vi "SP Build Key Array for Config.vi"(8 "error in (no error)":errorcluster, 9 "S Parameter Test Parameters":T2={"Stimulus"={"Use Instrument Settings"=FALSE, "Blank Frequencies"=FALSE, "Sweep Type"=enum."Linear", "Sweep"={"Fstart"=500.0, "Fstop"=1500.0, "Units"=enum."MHz", "Points"=2}, "Power (dBm)"=999.0, "IFBW (Hz)"=-1.0, "Sweep Time (s)"=-1.0, "Calibration"={"State"=FALSE, "String"=""}}, "Measurement"={"Auto Select"=TRUE, "Data Source"=enum."VNA", "Ports"=2, "Parameters"=[]}, "De-Embed"={"De-Embed"=FALSE, "Adapters"=[]}, "Display"={"Lock Control"=FALSE, "Retain Settings"=TRUE, "Formatted Data"=FALSE, "Plot Orientation"=enum."Single", "Plot Controls"=[{"Trace Orientation"=enum."Overlay", "Frequency"={"Change Frequency"=FALSE, "Start"=500.0, "Stop"=1500.0, "Units"=enum."MHz"}, "Markers"=[], "Traces"=[]}, {"Trace Orientation"=enum."Overlay", "Frequency"={"Change Frequency"=FALSE, "Start"=500.0, "Stop"=1500.0, "Units"=enum."MHz"}, "Markers"=[], "Traces"=[]}, {"Trace Orientation"=enum."Overlay", "Frequency"={"Change Frequency"=FALSE, "Start"=500.0, "Stop"=1500.0, "Units"=enum."MHz"}, "Markers"=[], "Traces"=[]}, {"Trace Orientation"=enum."Overlay", "Frequency"={"Change Frequency"=FALSE, "Start"=500.0, "Stop"=1500.0, "Units"=enum."MHz"}, "Markers"=[], "Traces"=[]}]}, "Limits"=[], "Filter Limits"=[]} {"Filter Limits"."Parameter"."Stimulus Port" min=1 step=1; "Filter Limits"."Parameter"."Response Port" min=1 step=1; "Filter Limits"."Passband"."Bandwidth Attn" format="%.3g"; "Filter Limits"."Passband"."Stop/Span" format="%.3g"; "Filter Limits"."Passband"."Start/Center" format="%.3g"; "Measurement"."Parameters"."Channel" min=0 max=32 step=1; "Measurement"."Parameters"."Parameter"."Stimulus Port" min=1 step=1; "Measurement"."Parameters"."Parameter"."Response Port" min=1 step=1; "Limits"."Parameter"."Stimulus Port" min=1 step=1; "Limits"."Parameter"."Response Port" min=1 step=1; "Stimulus"."Sweep Time (s)" format="%.3g"; "Display"."Plot Controls"."Traces"."Reference" format="%#.2g"; "Display"."Plot Controls"."Traces"."Display Data" items=["Data", "Memory", "Data/Memory"]; "Display"."Plot Controls"."Traces"."Format" items=["Log Mag", "Phase", "Expanded Phase", "Delay", "Smith", "Polar", "Lin Mag", "SWR", "Loss", "Real", "Imaginary"]; "Display"."Plot Controls"."Traces"."Scale" min=0.001 step=1.0 format="%#.2g"; "Display"."Plot Controls"."Traces"."Position" min=0.0 max=10.0; "Display"."Plot Controls"."Frequency"."Stop" format="%.3g"; "Display"."Plot Controls"."Frequency"."Start" format="%.3g"}, 10 "Key Array In":T33, 11 "Connection Refnum":T1) -> (0 "error out":errorcluster, 1 "$$INITCODE$$":string, 2 "Key Array Out":T33, 3 "Connection Refnum":T1)   [LabVIEW 2011]
uses:
  ITK EXT/utils/keyedarr.llb/Keyed Array.ctl
  TypeDefs/SP Test Parameters.ctl
  TypeDefs/SP Stimulus Parameters.ctl
  TypeDefs/SP Frequency Units.ctl
  TypeDefs/SP Calibration State.ctl
  TypeDefs/SP Measurement.ctl
  TypeDefs/SP Parameters.ctl
  TypeDefs/SP Parameter.ctl
  TypeDefs/SP De-Embed.ctl
  TypeDefs/SP Adapter.ctl
  TypeDefs/SP Data.ctl
  TypeDefs/SP Display Parameters.ctl
  TypeDefs/SP Display Plot Controls Cluster.ctl
  TypeDefs/SP Marker Cluster.ctl
  TypeDefs/SP Marker Type.ctl
  TypeDefs/SP Display Trace Controls.ctl
  TypeDefs/SP Display Format.ctl
  TypeDefs/SP Display Data.ctl
  TypeDefs/SP Limit.ctl
  TypeDefs/SP Format.ctl
  TypeDefs/SP Limit Type.ctl
  TypeDefs/SP Limit Point.ctl
  Test Referential Limit.ctl
  TypeDefs/SP Filter.ctl
  TypeDefs/SP Filter Type.ctl
  TypeDefs/SP Filter Passband.ctl
  TypeDefs/SP Frequency Format.ctl
  TypeDefs/SP Filter Ripple.ctl
  TypeDefs/SP Attenuation Point.ctl
  TypeDefs/SP Attenuation Type.ctl
  TypeDefs/SP Skirt Rejection Point.ctl
  TypeDefs/SP Relative Loss.ctl
  Summitek EXT/ODBC/SQL Controls/Connection Refnum.ctl
  ITK EXT/utils/strutil.llb/Case Matching.ctl
panel:
  # "Div"
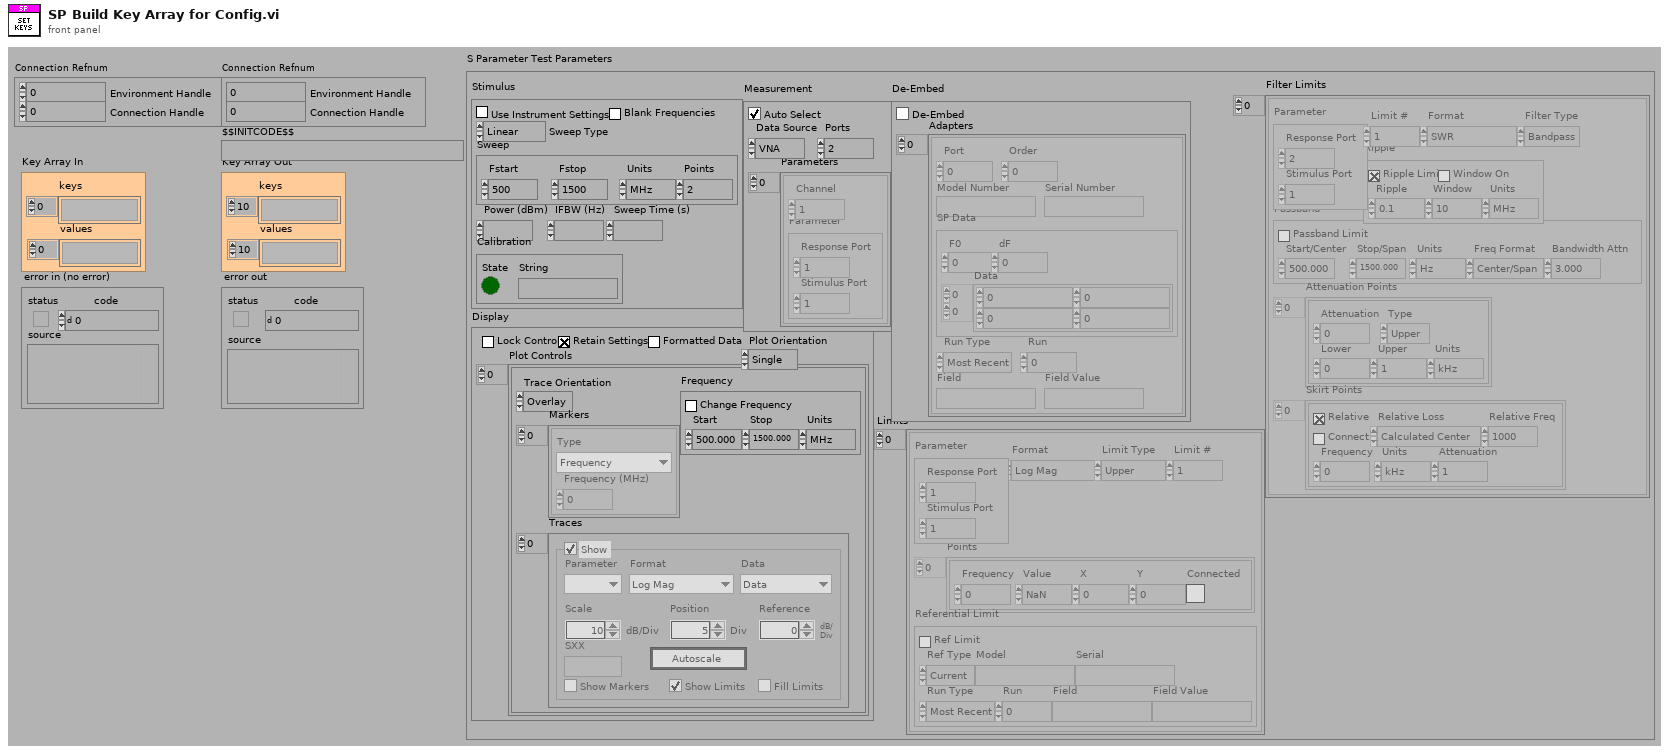
[diagram p1: front panel]
types:
  T1 = typedef "Connection Refnum.ctl" = cluster{"Environment Handle":i32, "Connection Handle":i32}
  T2 = typedef "SP Test Parameters.ctl" = cluster{"Stimulus":T3, "Measurement":T6, "De-Embed":T9, "Display":T12, "Limits":T19[], "Filter Limits":T24[]}
  T3 = typedef "SP Stimulus Parameters.ctl" = cluster{"Use Instrument Settings":bool, "Blank Frequencies":bool, "Sweep Type":enum32{"Linear", "Logarithmic", "List", "Power", "CW"}, "Sweep":cluster{"Fstart":dbl, "Fstop":dbl, "Units":T4, "Points":i32}, "Power (dBm)":dbl, "IFBW (Hz)":dbl, "Sweep Time (s)":dbl, "Calibration":T5}
  T4 = typedef "SP Frequency Units.ctl" = enum16{"Hz", "kHz", "MHz", "GHz", "Points"}
  T5 = typedef "SP Calibration State.ctl" = cluster{"State":bool, "String":string}
  T6 = typedef "SP Measurement.ctl" = cluster{"Auto Select":bool, "Data Source":enum16{"VNA", "Data File"}, "Ports":i8, "Parameters":T7[]}
  T7 = typedef "SP Parameters.ctl" = cluster{"Channel":i8, "Parameter":T8}
  T8 = typedef "SP Parameter.ctl" = cluster{"Stimulus Port":i8, "Response Port":i8}
  T9 = typedef "SP De-Embed.ctl" = cluster{"De-Embed":bool, "Adapters":T10[]}
  T10 = typedef "SP Adapter.ctl" = cluster{"Port":i8, "Order":i8, "Model Number":string, "Serial Number":string, "SP Data":T11, "Run Type":enum16{"Most Recent", "Run #", "Match Field"}, "Run":i32, "Field":string, "Field Value":string}
  T11 = typedef "SP Data.ctl" = cluster{"F0":dbl, "dF":dbl, "Data":cdb[][]}
  T12 = typedef "SP Display Parameters.ctl" = cluster{"Lock Control":bool, "Retain Settings":bool, "Formatted Data":bool, "Plot Orientation":enum32{"Single", "Dual", "Quad"}, "Plot Controls":T13[]}
  T13 = typedef "SP Display Plot Controls Cluster.ctl" = cluster{"Trace Orientation":enum32{"Overlay", "Split"}, "Frequency":cluster{"Change Frequency":bool, "Start":dbl, "Stop":dbl, "Units":T4}, "Markers":T14[], "Traces":T16[]}
  T14 = typedef "SP Marker Cluster.ctl" = cluster{"Type":T15, "Frequency (MHz)":dbl}
  T15 = typedef "SP Marker Type.ctl" = enum16{"Frequency", "Trace Maximum", "Trace Minimum", "Limit Maximum", "Limit Minimum"}
  T16 = typedef "SP Display Trace Controls.ctl" = cluster{"Trace On":bool, "Measure":i32, "Format":T17, "Autoscale":bool, "Reference":dbl, "\nRefUnit":string, "Position":dbl, "Scale":dbl, "ScaleUnit":string, "LimitOn":bool, "LimitFill":bool, "Display Data":T18, "Show Markers":bool, "SXX":string}
  T17 = typedef "SP Display Format.ctl" = i32
  T18 = typedef "SP Display Data.ctl" = u16
  T19 = typedef "SP Limit.ctl" = cluster{"Parameter":T8, "Format":T20, "Limit Type":T21, "Points":T22[], "Referential Limit":T23, "Limit #":i8}
  T20 = typedef "SP Format.ctl" = enum16{"Log Mag", "Lin Mag", "SWR", "Phase", "Expanded Phase", "Delay", "Insertion Loss", "Isolation", "Return Loss"}
  T21 = typedef "SP Limit Type.ctl" = enum16{"Upper", "Lower", "Delta", "Filter", "Referential"}
  T22 = typedef "SP Limit Point.ctl" = cluster{"Frequency":dbl, "Value":dbl, "X":dbl, "Y":dbl, "Connected":bool}
  T23 = typedef "Test Referential Limit.ctl" = cluster{"Ref Limit":bool, "Ref Type":enum16{"Current", "Specify"}, "Model":string, "Serial":string, "Run Type":enum16{"Most Recent", "Run #", "Match Field"}, "Run":i32, "Field":string, "Field Value":string}
  T24 = typedef "SP Filter.ctl" = cluster{"Limit #":i8, "Parameter":T8, "Format":T20, "Filter Type":T25, "Passband":T26, "Ripple":T28, "Attenuation Points":T29[], "Skirt Points":T31[]}
  T25 = typedef "SP Filter Type.ctl" = enum16{"Lowpass", "Highpass", "Bandpass", "Bandstop"}
  T26 = typedef "SP Filter Passband.ctl" = cluster{"Start/Center":dbl, "Stop/Span":dbl, "Units":T4, "Freq Format":T27, "Bandwidth Attn":dbl, "Passband Limit":bool}
  T27 = typedef "SP Frequency Format.ctl" = enum16{"Start/Stop", "Center/Span"}
  T28 = typedef "SP Filter Ripple.ctl" = cluster{"Ripple Limit":bool, "Window On":bool, "Ripple":dbl, "Window":dbl, "Units":T4}
  T29 = typedef "SP Attenuation Point.ctl" = cluster{"Attenuation":dbl, "Type":T30, "Lower":dbl, "Upper":dbl, "Units":T4}
  T30 = typedef "SP Attenuation Type.ctl" = enum16{"Center", "Lower", "Upper"}
  T31 = typedef "SP Skirt Rejection Point.ctl" = cluster{"Relative":bool, "Connect":bool, "Frequency":dbl, "Units":T4, "Attenuation":dbl, "Relative Loss":T32, "Relative Freq":dbl}
  T32 = typedef "SP Relative Loss.ctl" = enum16{"Calculated Center", "Passband Minimum", "Passband Maximum", "Passband Average", "Frequency"}
  T33 = typedef "Keyed Array.ctl" = cluster{"keys":string[], "values":string[]}
  T34 = typedef "Case Matching.ctl" = enum16{"a != A", "a == A", "system"}
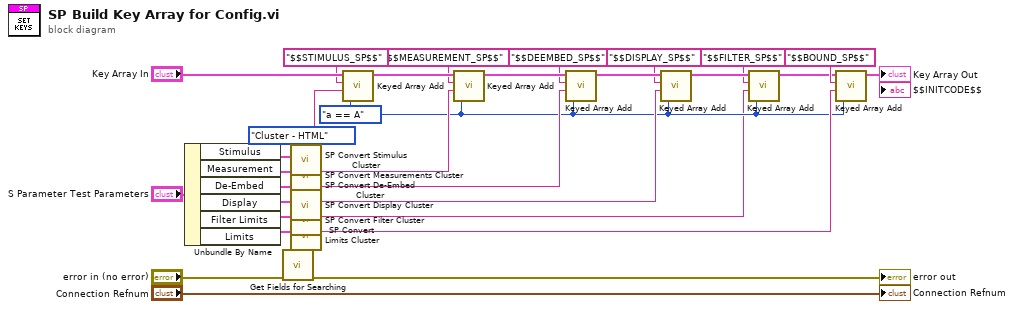
[diagram p0: block diagram]
diagram:
  w5 = Case_Matching."a == A" ("case matching (sensitive)")
  w3 = enum16{"Cluster - HTML", "HTML - Cluster"}."Cluster - HTML" ("Conversion")
  n1 = Unbundle By Name("S Parameter Test Parameters") -> ("Stimulus"=w16:T3, "Measurement"=w15:T6, "De-Embed"=w12:T9, "Display"=w26:T12, "Filter Limits"=w2:T24[], "Limits"=w27:T19[])
  n2 = call "Get Fields for Searching.vi"("error in"="error in (no error)") -> ("error out"=→"error out":errorcluster, "Field Records List"=w1:string[])  [unwired: 9 out]
  n3 = call "SP Convert Stimulus Cluster.vi"("Conversion"=w3, "Stimulus Cluster In"=w16) -> ("Stimulus HTML Out"=w23:string)  [unwired: 1 in, 5 out]
  n4 = call "SP Convert Measurements Cluster.vi"("Conversion"=w3, "Measurements Cluster In"=w15) -> ("Measurements HTML Out"=w21:string)  [unwired: 1 in, 5 out]
  n5 = call "SP Convert De-Embed Cluster.vi"("Fields Names"=w1, "Conversion"=w3, "De-Embed Cluster In"=w12) -> ("Measurements HTML Out"=w13:string)  [unwired: 1 in, 5 out]
  n6 = call "SP Convert Display Cluster.vi"("Conversion"=w3, "Display Cluster In"=w26) -> ("Display HTML Out"=w19:string)  [unwired: 1 in, 5 out]
  n7 = call "SP Convert Filter Cluster.vi"("Conversion"=w3, "Filter Cluster In"=w2) -> ("Filter HTML Out"=w4:string)  [unwired: 1 in, 6 out]
  n8 = call "SP Convert Limits Cluster.vi"("Fields Names"=w1, "Conversion"=w3, "Limits Cluster In"=w27) -> ("Limits HTML Out"=w17:string)  [unwired: 1 in, 5 out]
  n9 = call "Keyed Array Add.vi"("case matching (sensitive)"=w5, "value"=w23, "key"="$$STIMULUS_SP$$", "array in"="Key Array In") -> ("array out"=w29:T33)  [unwired: 3 out]
  n10 = call "Keyed Array Add.vi"("case matching (sensitive)"=w5, "value"=w21, "key"="$$MEASUREMENT_SP$$", "array in"=w29) -> ("array out"=w32:T33)  [unwired: 3 out]
  n11 = call "Keyed Array Add.vi"("case matching (sensitive)"=w5, "value"=w13, "key"="$$DEEMBED_SP$$", "array in"=w32) -> ("array out"=w31:T33)  [unwired: 3 out]
  n12 = call "Keyed Array Add.vi"("case matching (sensitive)"=w5, "value"=w19, "key"="$$DISPLAY_SP$$", "array in"=w31) -> ("array out"=w8:T33)  [unwired: 3 out]
  n13 = call "Keyed Array Add.vi"("case matching (sensitive)"=w5, "value"=w4, "key"="$$FILTER_SP$$", "array in"=w8) -> ("array out"=w7:T33)  [unwired: 3 out]
  n14 = call "Keyed Array Add.vi"("case matching (sensitive)"=w5, "value"=w17, "key"="$$BOUND_SP$$", "array in"=w7) -> ("array out"=→"Key Array Out":T33)  [unwired: 3 out]
  "Connection Refnum" <- "Connection Refnum"
